vi "GetQualifiedHierarchy.vi"(8 "error in (no error)":errorcluster, 11 "CLabVIEWItem in":refnum<class "CLabVIEWItem.lvclass">) -> (0 "error out":errorcluster, 1 "Qualified hierarchy":string[](array[string]), 3 "CLabVIEWItem out":refnum<class "CLabVIEWItem.lvclass">)   [LabVIEW 2020, in "LabVIEWItem.lvlib" / "CLabVIEWItem.lvclass"]
uses:
  CLabVIEWItem.lvclass
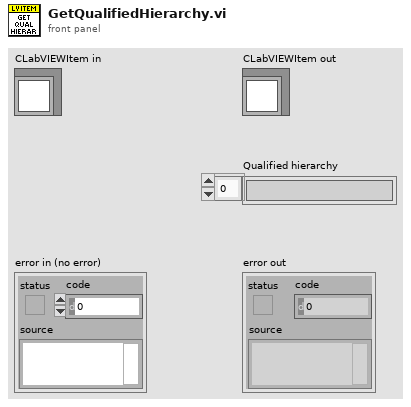
[diagram p1: front panel]
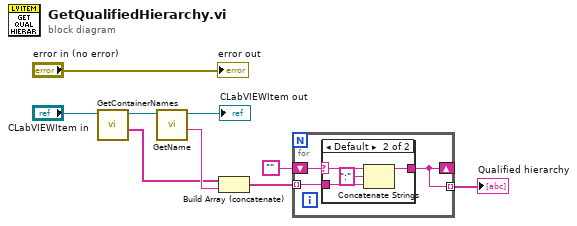
[diagram p0: block diagram]
diagram:
  n1 = call-dynamic "GetContainerNames.vi"("CLabVIEWItem in"="CLabVIEWItem in") -> ("Container name[]"=w3:string[], "CLabVIEWItem out"=w8:refnum<class "CLabVIEWItem.lvclass">)  [unwired: 8 in, 1 out]
  n2 = call-dynamic "GetName.vi"("CLabVIEWItem in"=w8) -> ("Name"=w4:string, "CLabVIEWItem out"=→"CLabVIEWItem out":refnum<class "CLabVIEWItem.lvclass">)  [unwired: 8 in, 1 out]
  n3 = Build Array (concatenate)(w3, w4) -> (w2:string[])
  n4 = for {
    tunnel: w2 -> [w12] mode=indexing
    shift-right: [w10] -> _
    shift-left: "" -> [w11]
    tunnel: [w10] -> w1 mode=indexing
    n5 = case shown="Default" w11 {
      selector: w11 -> [_ w14]
      tunnel: w12 -> [w13 w16]
      tunnel: [w13 w15] -> w10
      frame "" {
      }
      frame Default {
        n6 = Concatenate Strings(w14, ":" ("string"), w16) -> (w15:string)
      }
    }
  }
  "Qualified hierarchy" <- w1
  "error out" <- "error in (no error)"
